vi "SwitchPostCheck.vi"(7 "switch_data_array":T1(array[cluster]), 9 "Max Distance":dbl=20.0 format="%#_13g", 11 "All Lines in":T2) -> ()   [LabVIEW 2014, in "Map Data.lvlib"]
uses:
  Map Data.lvlib
  All-Lines.ctl
  LineCluster.ctl
  LineConnection.ctl
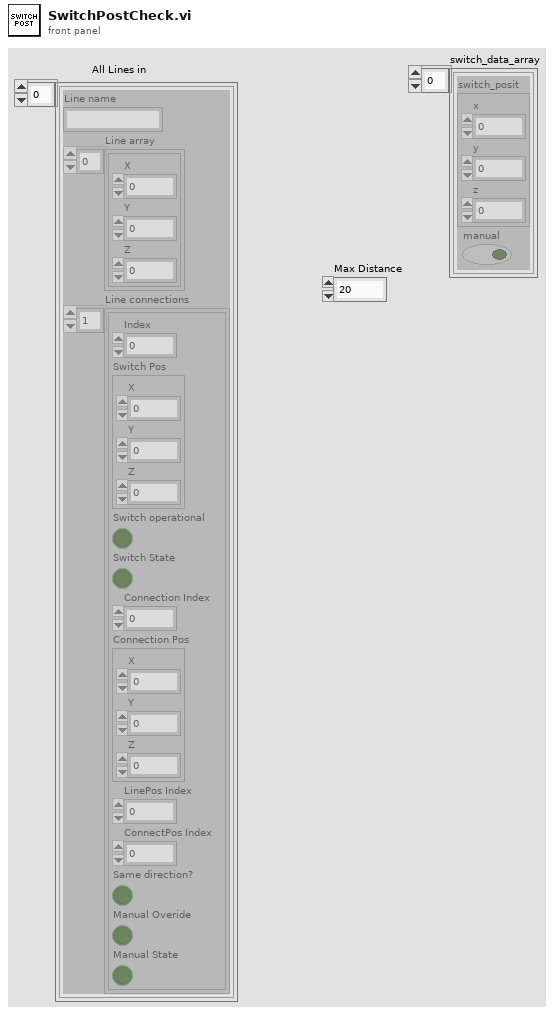
[diagram p1: front panel]
types:
  T1 = cluster{"switch_posit":cluster{"x":dbl, "y":dbl, "z":dbl}, "manual":bool}[]
  T2 = typedef "Map Data.lvlib/All-Lines.ctl" = T3[]
  T3 = typedef "Map Data.lvlib/LineCluster.ctl" = cluster{"Line name":string, "Line array":cluster{"X":dbl, "Y":dbl, "Z":dbl}[], "Line connections":T4[]}
  T4 = typedef "Map Data.lvlib/LineConnection.ctl" = cluster{"Index":i32, "Switch Pos":cluster{"X":dbl, "Y":dbl, "Z":dbl}, "Switch operational":bool, "Switch State":bool, "Connection Index":i32, "Connection Pos":cluster{"X":dbl, "Y":dbl, "Z":dbl}, "LinePos Index":i32, "ConnectPos Index":i32, "Same direction?":bool, "Manual Overide":bool, "Manual State":bool}
  T5 = cluster{"train_control_array":cluster{"uuid":string, "throttle":dbl, "brake":dbl, "horn":dbl, "wait":dbl, "name":string, "mode":string, "dest":string}[], "switch_control_array":cluster{"switch_posit":cluster{"x":dbl, "y":dbl, "z":dbl}, "switch":bool, "invert":bool, "wait":dbl}[]}
  T6 = cluster{"switch_posit":cluster{"x":dbl, "y":dbl, "z":dbl}, "switch":bool, "invert":bool, "wait":i32}
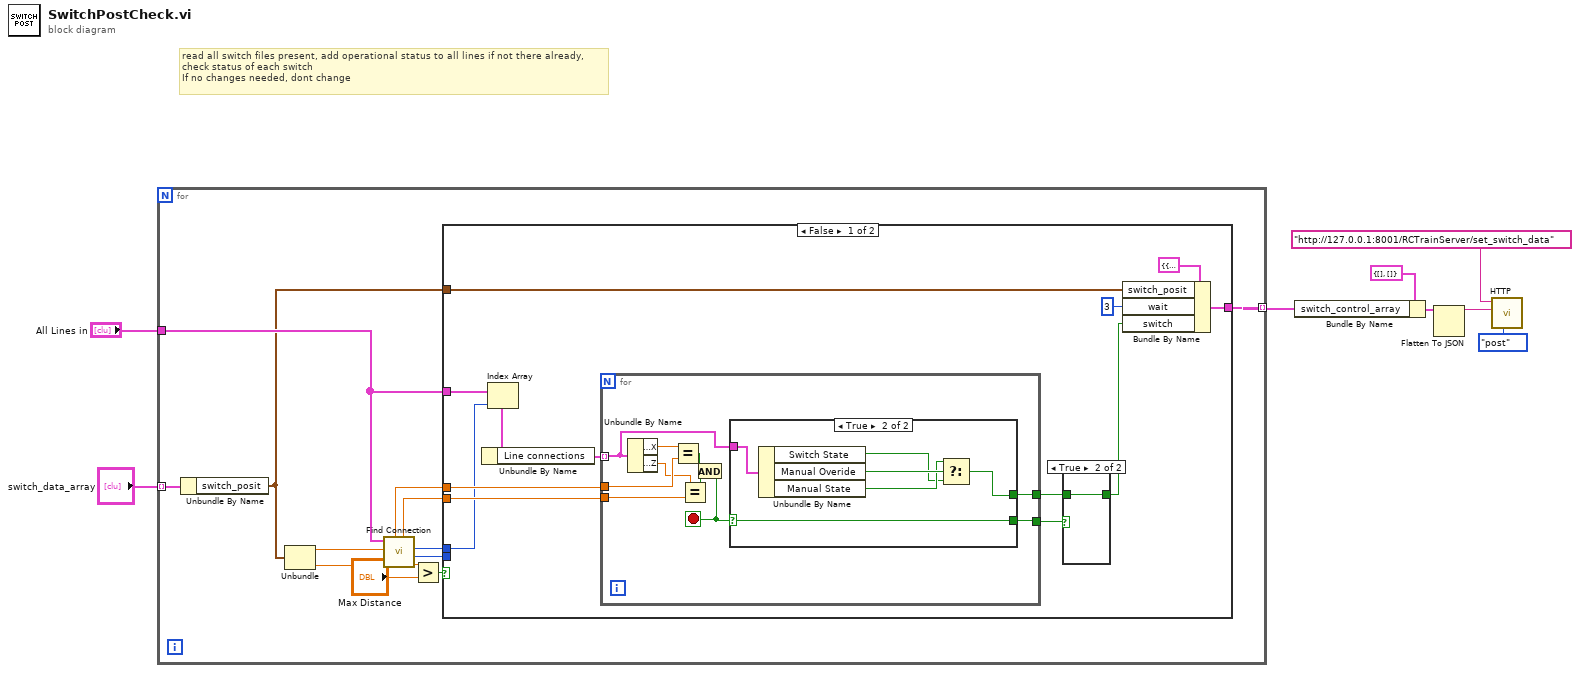
[diagram p0: block diagram]
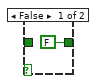
[diagram p2: hidden frame]
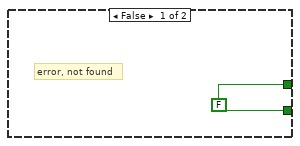
[diagram p3: hidden frame]
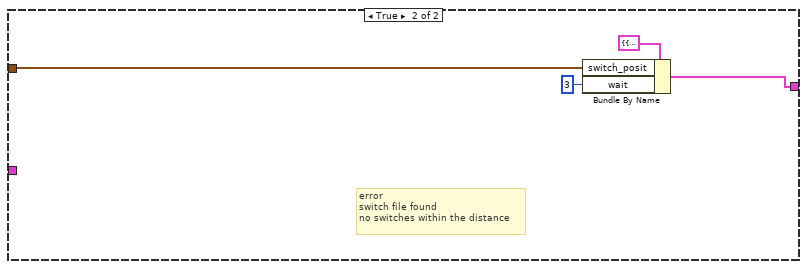
[diagram p4: hidden frame]
diagram:
  # "read all switch files present, add operational status to all lines if not there already,\ncheck status of each switch\nIf no changes needed, dont change"
  n1 = for {
    tunnel: "All Lines in" -> [w21]
    tunnel: "switch_data_array" -> [w20] mode=indexing
    tunnel: [w9] -> w1 mode=indexing
    n2 = Unbundle By Name(w20) -> ("switch_posit"=w10:cluster{"x":dbl, "y":dbl, "z":dbl})
    n3 = Unbundle(w10) -> ("x"=w19:dbl, "z"=w18:dbl)  [unwired: 1 out]
    n4 = call "Find Connection.vi"("Z"=w18, "X"=w19, "All Lines"=w21) -> ("Distance to nearest"=w17:dbl, "Index on Line"=w14:i32, "Nearest Line"=w13:i32, "Z Coonnection"=w12:dbl, "X Connection"=w11:dbl)  [unwired: 2 in, 2 out]
    n5 = Greater?(x=w17, y="Max Distance") -> (0:w16:bool)
    n6 = case shown="False" w16 {
      tunnel: w14 -> [_ _]
      tunnel: w13 -> [w29 _]
      tunnel: w21 -> [w34 _]
      tunnel: w12 -> [w31 _]
      tunnel: w11 -> [w32 _]
      tunnel: w10 -> [w23 w55]
      tunnel: [w22 w54] -> w9
      frame False {
        n7 = Index Array(array=w34, index=w29) -> (element=w30:T3)
        n8 = Unbundle By Name(w30) -> ("Line connections"=w33:T4[])
        n9 = for {
          tunnel: w33 -> [w40] mode=indexing
          tunnel: w32 -> [w45]
          tunnel: w31 -> [w43]
          tunnel: [w38] -> w28
          tunnel: [w37] -> w26
          stop <- w39 stop-if-true
          n10 = Unbundle By Name(w40) -> ("Switch Pos.X"=w46:dbl, "Switch Pos.Z"=w44:dbl)
          n11 = Equal?(x=w46, y=w45) -> (x = y?=w42:bool)
          n12 = Equal?(x=w44, y=w43) -> (x = y?=w41:bool)
          n13 = And(x=w42, y=w41) -> (x .and. y?=w39:bool)
          n14 = case shown="True" w39 {
            selector: w39 -> [_ w53]
            tunnel: w40 -> [_ w52]
            tunnel: [w47 w53] -> w38
            tunnel: [w47 w48] -> w37
            frame False {
              w47 = FALSE
              # "error, not found"
            }
            frame True {
              n15 = Unbundle By Name(w52) -> ("Switch State"=w49:bool, "Manual Overide"=w51:bool, "Manual State"=w50:bool)
              n16 = Select(t=w50, s=w51, f=w49) -> (s? t:f=w48:bool)
            }
          }
        }
        n17 = case shown="True" w28 {
          tunnel: w26 -> [_ w36]
          tunnel: [FALSE ("Switch State") w36] -> w25
          frame False {
          }
          frame True {
          }
        }
        n18 = Bundle By Name(cluster=T6 {"switch_posit"={"x"=0.0, "y"=0.0, "z"=0.0}, "switch"=FALSE, "invert"=FALSE, "wait"=0} ("switch_control"), "switch_posit"=w23, "wait"=3, "switch"=w25) -> (w22:T6)
      }
      frame True {
        # "error\nswitch file found\nno switches within the distance"
        n19 = Bundle By Name(cluster=T6 {"switch_posit"={"x"=0.0, "y"=0.0, "z"=0.0}, "switch"=FALSE, "invert"=FALSE, "wait"=0} ("switch_control"), "switch_posit"=w55, "wait"=3) -> (w54:T6)
      }
    }
  }
  n20 = Bundle By Name(cluster=T5 {"train_control_array"=[], "switch_control_array"=[]} ("output cluster"), "switch_control_array"=w1) -> (w6:T5)
  n21 = Flatten To JSON(anything=w6) -> (JSON string=w4:string)  [unwired: 2 in, 1 out]
  n22 = call "HTTP.vi"("Enum"=enum16{"close", "post", "get", "init"}."post", "data in"=w4, "url"="http://127.0.0.1:8001/RCTrainServer/set_switch_data") -> ()  [unwired: 7 in, 2 out]
